vi "pointReactorSimulator.vi"() -> ()   [LabVIEW 2020]
doc: "本程序通过点堆动力学模型模拟核电站的反应堆运行状态。"
uses:
  <vilib>/Utility/sysdir.llb/System Directory Type.ctl
  <vilib>/NI/Modbus Library/API/Slave/Modbus Slave.lvclass
  <vilib>/Utility/error.llb/DialogType.ctl
  Keithley 622x/Utility/Typedefs/KE622x -- Instrument Type.ctl
  Keithley 622x/Configure/Source/Typedefs/KE622x -- Voltage Limit.ctl
  Keithley 622x/Configure/Source/Typedefs/KE622x -- Current Range.ctl
  Keithley 622x/Configure/Source/Typedefs/KE622x -- Current Ranges.ctl
  <vilib>/DAQmx/write.llb/DAQmx Write (Counter 1D Frequency 1Chan NSamp).vi
  <vilib>/DAQmx/write.llb/DAQmx Write (Analog DBL 1Chan 1Samp).vi
  SettingVariable.vi
  <vilib>/Utility/file.llb/Read Delimited Spreadsheet (DBL).vi
  <userlib>/_OpenG.lib/array/array.llb/Reverse 2D Array (DBL)__ogtk.vi
  <vilib>/Analysis/polynomials.llb/Scalar Polynomial Evaluation (DBL).vi
  <vilib>/NI/Modbus Library/API/Wrapper/Create TCP Slave.vi
  <vilib>/Instr/_visa.llb/VISA Configure Serial Port (Instr).vi
  <vilib>/DAQmx/create/channels.llb/DAQmx Create Channel (CO-Pulse Generation-Frequency).vi
  <vilib>/DAQmx/configure/timing.llb/DAQmx Timing (Implicit).vi
  <vilib>/DAQmx/create/channels.llb/DAQmx Create Channel (AO-Voltage-Basic).vi
  <vilib>/DAQmx/miscellaneous.llb/DAQmx Fill In Error Info.vi
  PointReactorDll.dll
  <vilib>/Analysis/NI_AALPro.lvlib
  Keithley 622x/Keithley 622x.lvlib
  <vilib>/NI/Modbus Library/API/Wrapper/API Main.lvlib
panel:
  in  "退出":bool
  out "KE6220_2":bool
  in  "物理参数设置":bool
  out "反应性仪输出电压":dbl[](array[numeric])
  out "输出电压":dbl[](array[numeric])
  in  "输出电流 (A)":dbl
  in  "电压输出选择":bool
  out "中子注量率":dbl caption="(n/cm2·s)"
  out "硼总价值 (pcm)":dbl
  out "棒总价值 (pcm)":dbl
  out "硼浓度 indicator":dbl
  in  "硼浓度 (ppm)":dbl(slide)=1.0 scale=0.0..2000.0
  out "运行时间":dbl caption="(s)"
  in  "TCP端口号":u16=502 caption="TCP端口号：" min=1 max=9999
  out "堆芯反应性(硼+棒) (pcm)":dbl
  out "keff":dbl
  in  "S棒组":dbl(slide)=200.0 min=0.0 max=225.0 scale=0.0..225.0
  in  "A棒组":dbl(slide)=200.0 min=0.0 max=225.0 scale=0.0..225.0
  in  "B棒组":dbl(slide)=200.0 min=0.0 max=225.0 scale=0.0..225.0
  in  "C棒组":dbl(slide)=200.0 min=0.0 max=225.0 scale=0.0..225.0
  in  "堆芯后备反应性 (pcm)":dbl
  out "S棒价值":dbl
  out "A棒价值":dbl
  out "B棒价值":dbl
  out "C棒价值":dbl
  out "D棒价值":dbl
  out "中子注量曲线":dbl(graph) caption="波形图"
  in  "D棒组":dbl(slide)=200.0 min=0.0 max=225.0 scale=0.0..225.0
  out "CARD":bool
  out "KE6220_1":bool
  out "COM2":bool
  out "COM1":bool
  in  "VO 4":u16(ring)=3 items=["D棒位 (step)", "C棒位 (step)", "B棒位 (step)", "A棒位 (step)", "S棒位 (step)", "硼浓度 (ppm)", "中间量程电流 (A)", "源量程计数 (CPS)"]
  in  "VO 3":u16(ring)=2 items=["D棒位 (step)", "C棒位 (step)", "B棒位 (step)", "A棒位 (step)", "S棒位 (step)", "硼浓度 (ppm)", "中间量程电流 (A)", "源量程计数 (CPS)"]
  in  "VO 2":u16(ring)=1 items=["D棒位 (step)", "C棒位 (step)", "B棒位 (step)", "A棒位 (step)", "S棒位 (step)", "硼浓度 (ppm)", "中间量程电流 (A)", "源量程计数 (CPS)"]
  in  "VO 1":u16(ring) items=["D棒位 (step)", "C棒位 (step)", "B棒位 (step)", "A棒位 (step)", "S棒位 (step)", "硼浓度 (ppm)", "中间量程电流 (A)", "源量程计数 (CPS)"]
  in  "电信号输出设置":bool
  in  "TCP服务器开关":bool caption="TCP服务器开："
  in  "电流输出选择":u16(ring) items=["中间量程电流", "功率量程电流"]
  out "棒位与硼浓度":dbl[](array[numeric])
  in  "反应性控制方式":bool
  in  "归零":bool
  in  "棒速(step/min)":dbl=72.0 min=1.0 max=10000.0 step=1.0 format="%#.3g"
  in  "开始降棒":bool
  in  "降棒选择":u16(ring) items=["D棒组", "C棒组", "B棒组", "A棒组", "S棒组"]
  in  "细分时间 (ms)":u32=100 min=10 max=1000 step=1
  in  "开始":bool
  in  "时间比例尺":dbl(knob)=1.0 min=0.1 max=1000.0 step=0.1 scale=0.1..1000.0
  out "功率量程 (A)":dbl(slide) scale=2.875e-12..0.00023 scale format="%#_6e"
  out "中间量程 (A)":dbl(slide) scale=1e-11..0.0008 scale format="%#_6e"
  out "源量程 (CPS)":dbl(slide) scale=1.0..1000000.0 scale format="%#_6f"
  out "%FP":dbl(slide) scale=2e-09..200.0 scale format="%#_6e"
  out "中子注量率":dbl(slide) scale=0.1..10000000000.0 scale format="%#_6e"
  in  "时间步长":dbl=0.1 caption="时间步长："
  in  "初始注量率":dbl=1000.0 caption="初始注量率：" format="%#_4g"
  in  "堆芯反应性":dbl caption="堆芯反应性 (pcm)"
  in  "停止":bool
  # "反应性仪测试用点堆模拟器"
  # "探测器"
  # "手输"
  # "棒硼"
  # "1.25E+5 n/cm2·s\n——"
  # "——\n1.25E+2 n/cm2·s"
  # "——  1.25E-1 n/cm2·s"
  # "(n/cm2·s)"
  # "硬件测试"
  # "(s)"
  # "0-10V"
  # "1-5V"
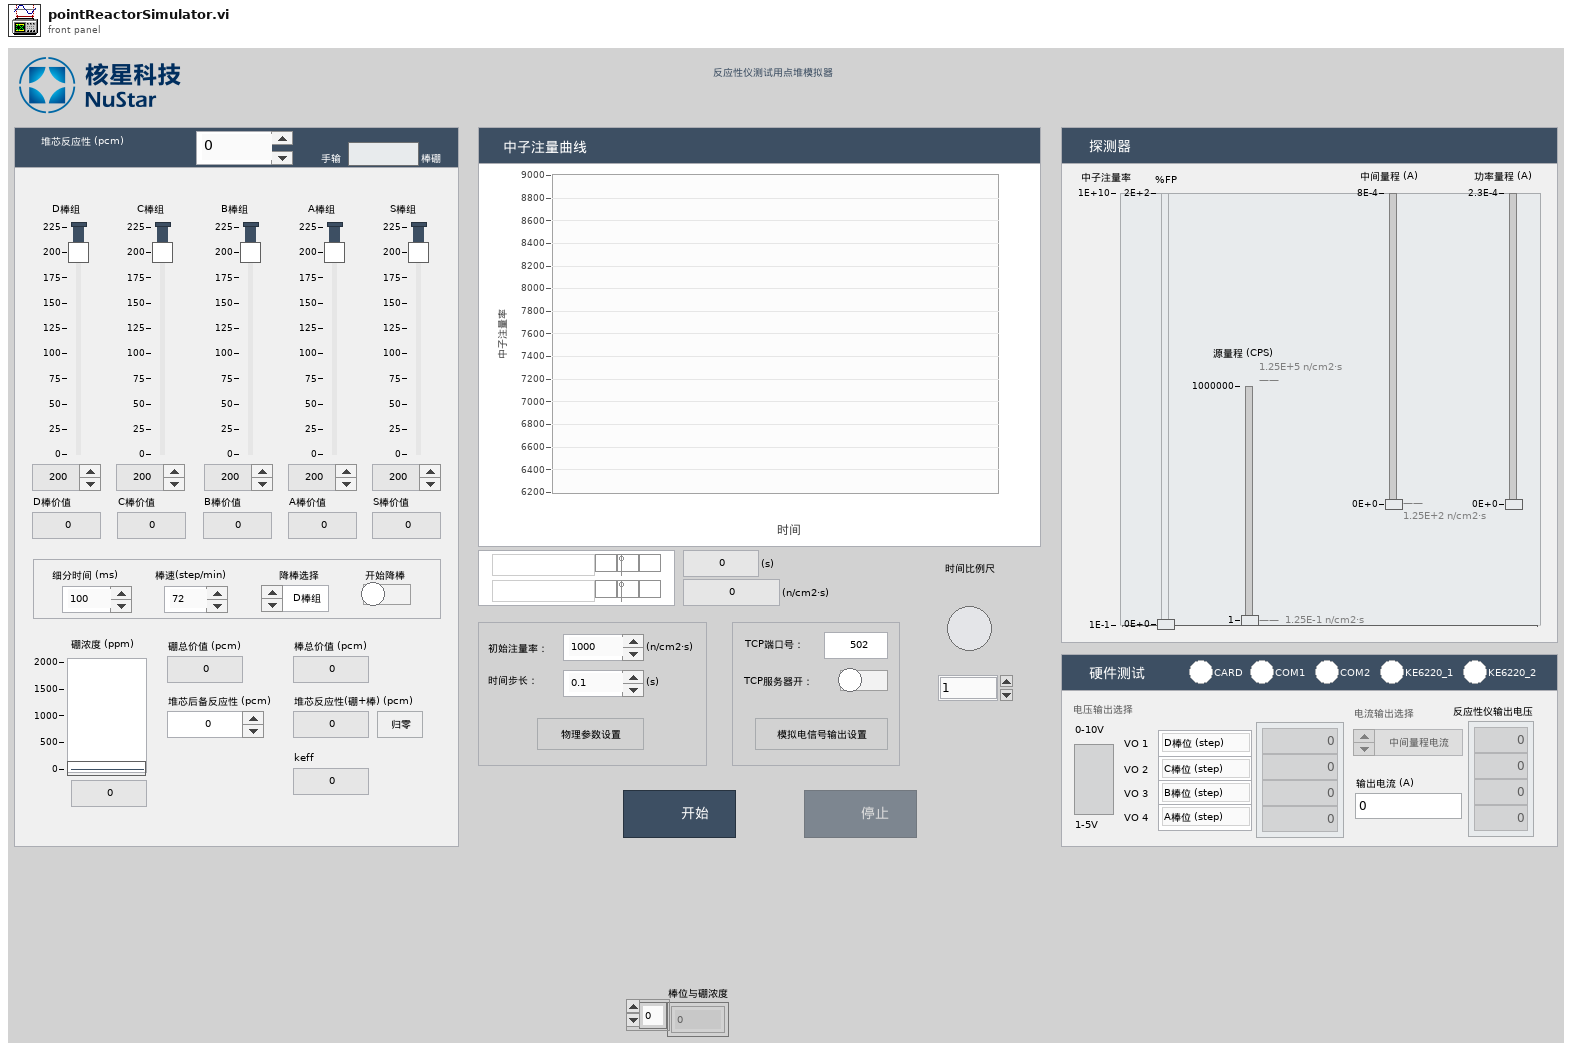
[diagram p1: front panel]
types:
  T1 = enum8{"Enabled", "Disabled", "Disabled and Grayed Out"}
  T2 = enum16{"open", "replace", "create", "open or create", "replace or create", "replace or create with confirmation"}
  T3 = typedef "Keithley 622x.lvlib/KE622x -- Voltage Limit.ctl" = dbl
  T4 = typedef "Keithley 622x.lvlib/KE622x -- Instrument Type.ctl" = enum16{"KE6220", "KE6221"}
  T5 = typedef "System Directory Type.ctl" = i32
  T6 = typedef "DialogType.ctl" = u16
  T7 = typedef "Keithley 622x.lvlib/KE622x -- Current Range.ctl" = cluster{"Auto Range?":bool, "Man / Selected\nRange":T8}
  T8 = typedef "Keithley 622x.lvlib/KE622x -- Current Ranges.ctl" = enum16{"2nA", "20nA", "200nA", "2uA", "20uA", "200uA", "2mA", "20mA", "100mA"}
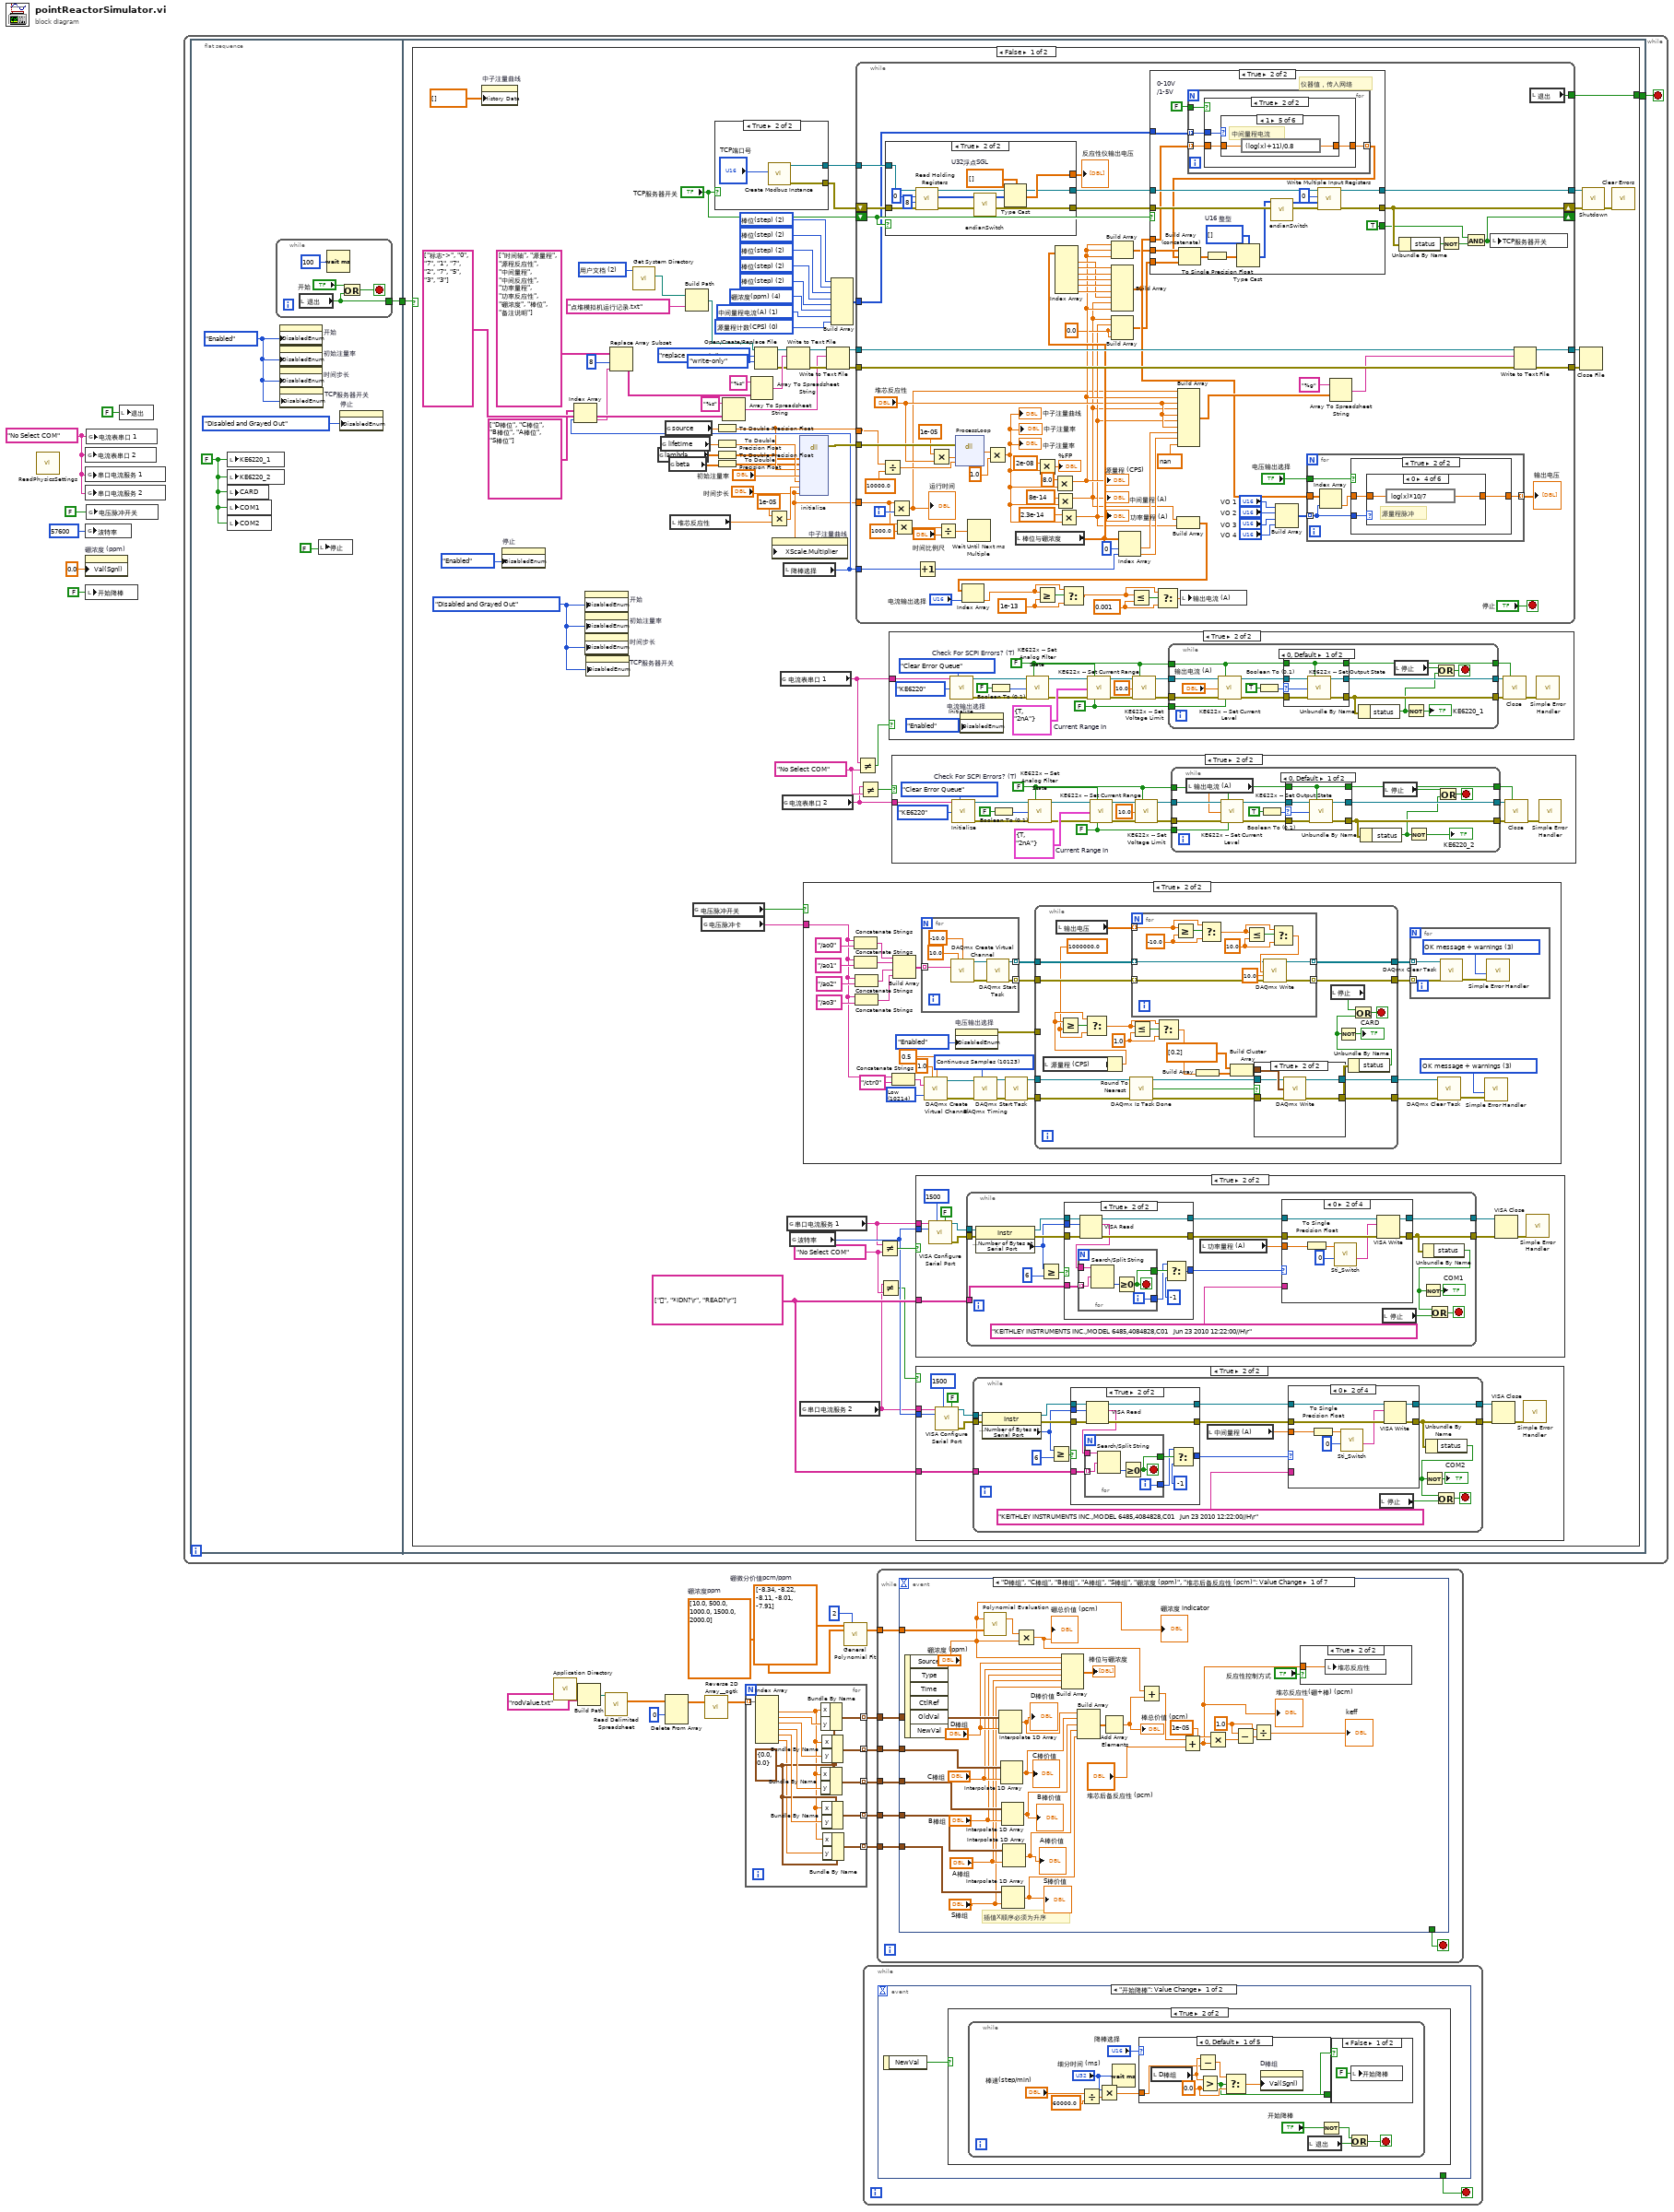
[diagram p0: block diagram]
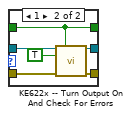
[diagram p3: hidden frame]
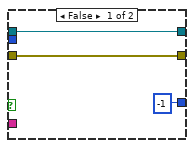
[diagram p5: hidden frame]
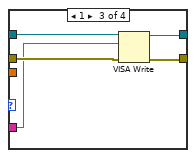
[diagram p7: hidden frame]
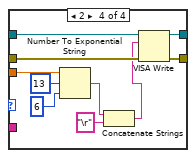
[diagram p8: hidden frame]
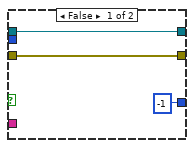
[diagram p10: hidden frame]
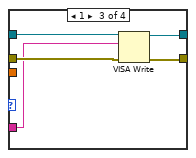
[diagram p12: hidden frame]
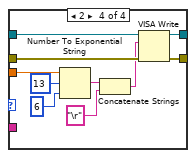
[diagram p13: hidden frame]
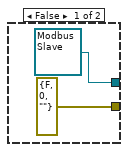
[diagram p14: hidden frame]
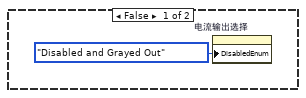
[diagram p15: hidden frame]
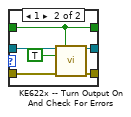
[diagram p16: hidden frame]
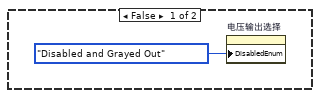
[diagram p17: hidden frame]
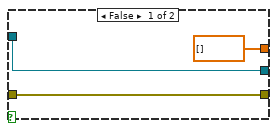
[diagram p19: hidden frame]
diagram:
  w12 = "No Select COM" ("新元素/子数组")
  w20 = dbl[] [-8.34, -8.22, -8.11, -8.01, -7.91]  # 硼微分价值pcm/ppm
  w19 = dbl[] [10.0, 500.0, 1000.0, 1500.0, 2000.0]  # 硼浓度ppm
  n1 = call "ReadPhysicsSettings.vi"() -> ()  [unwired: 12 in]
  n2 = property on="硼浓度 (ppm)" class="Slide (strict)"("Val(Sgnl)"=0.0 ("Value (Signaling)")) -> ()  [unwired: 2 in, 2 out]
  n3 = global write "SettingVariable.vi" "电流表串口 2"(w12) -> ()
  n4 = global write "SettingVariable.vi" "串口电流服务 1"(w12) -> ()
  n5 = global write "SettingVariable.vi" "串口电流服务 2"(w12) -> ()
  n6 = global write "SettingVariable.vi" "波特率"(u32 57600 ("波特率")) -> ()
  n7 = local write "开始降棒"(FALSE ("开始降棒")) -> ()
  n8 = global write "SettingVariable.vi" "电流表串口 1"(w12) -> ()
  n9 = global write "SettingVariable.vi" "电压脉冲开关"(FALSE ("电压脉冲开关")) -> ()
  n10 = local write "退出"(FALSE ("退出")) -> ()
  n11 = while {
    stop <- w24 stop-if-true
    n12 = flat-sequence {
      tunnel: [w26] -> w23
      tunnel: [w35] -> w24
      tunnel: w23 -> [w34]
      frame #0 {
        w29 = FALSE ("KE6220_1")
        w25 = T1."Enabled" ("禁用")
        n13 = local write "KE6220_1"(w29) -> ()
        n14 = local write "KE6220_2"(w29) -> ()
        n15 = local write "CARD"(w29) -> ()
        n16 = local write "COM1"(w29) -> ()
        n17 = local write "COM2"(w29) -> ()
        n18 = while {
          tunnel: [w30] -> w26
          stop <- w32 stop-if-true
          n19 = local read "退出"() -> (w30:bool)
          n20 = Wait (ms)(milliseconds to wait=u32 100) -> ()  [unwired: 1 out]
          n21 = Or(x="开始", y=w30) -> (x .or. y?=w32:bool)
        }
        n22 = property on="开始" class="Bool"("DisabledEnum"=w25) -> ()  [unwired: 2 in, 2 out]
        n23 = property on="初始注量率" class="DigNum (strict)"("DisabledEnum"=w25) -> ()  [unwired: 2 in, 2 out]
        n24 = property on="时间步长" class="DigNum (strict)"("DisabledEnum"=w25) -> ()  [unwired: 2 in, 2 out]
        n25 = property on="TCP服务器开关" class="Bool (strict)"("DisabledEnum"=w25) -> ()  [unwired: 2 in, 2 out]
        n26 = local write "停止"(FALSE ("退出")) -> ()
        n27 = property on="停止" class="Bool (strict)"("DisabledEnum"=T1."Disabled and Grayed Out" ("禁用")) -> ()  [unwired: 2 in, 2 out]
      }
      frame #1 {
        n28 = case shown="False" w34 {
          tunnel: [w47 TRUE ("退出")] -> w35
          frame False {
            w36 = T1."Disabled and Grayed Out" ("禁用")
            w67 = u16 0 items=["源量程计数(CPS)", "中间量程电流(A)", "棒位(step)", "温度(℃)", "硼浓度(ppm)", "P2电压信号"] ("P2-1")
            w68 = u16 1 items=["源量程计数(CPS)", "中间量程电流(A)", "棒位(step)", "温度(℃)", "硼浓度(ppm)", "P2电压信号"] ("P2-1")
            w69 = u16 4 items=["源量程计数(CPS)", "中间量程电流(A)", "棒位(step)", "温度(℃)", "硼浓度(ppm)", "P2电压信号"] ("P2-1")
            w70 = u16 2 items=["源量程计数(CPS)", "中间量程电流(A)", "棒位(step)", "温度(℃)", "硼浓度(ppm)", "P2电压信号"] ("P2-1")
            w71 = u16 2 items=["源量程计数(CPS)", "中间量程电流(A)", "棒位(step)", "温度(℃)", "硼浓度(ppm)", "P2电压信号"] ("P2-1")
            w72 = u16 2 items=["源量程计数(CPS)", "中间量程电流(A)", "棒位(step)", "温度(℃)", "硼浓度(ppm)", "P2电压信号"] ("P2-1")
            w73 = u16 2 items=["源量程计数(CPS)", "中间量程电流(A)", "棒位(step)", "温度(℃)", "硼浓度(ppm)", "P2电压信号"] ("P2-1")
            w57 = "No Select COM" ("新元素/子数组")
            w79 = T5 2 items=["用户目录"=0, "用户桌面"=1, "用户文档"=2, "用户应用程序数据"=3, "用户设置"=4, "用户临时目录"=5, "公共文档"=6, "公共应用程序数据"=7, "公共设置"=8, "公共缓存"=13, "系统核心库"=9, "系统安装库"=10, "应用程序文件"=11, "启动盘根目录"=12] ("system directory type")
            w81 = "No Select COM" ("新元素/子数组")
            w83 = string[] ["", "*IDN?\r", "READ?\r"] ("添加的数组")
            w85 = u16 2 items=["源量程计数(CPS)", "中间量程电流(A)", "棒位(step)", "温度(℃)", "硼浓度(ppm)", "P2电压信号"] ("P2-1")
            n29 = property on="中子注量曲线" class="WFChart (strict)"("History Data"=dbl[] []) -> ()  [unwired: 2 in, 2 out]
            n30 = property on="停止" class="Bool (strict)"("DisabledEnum"=T1."Enabled" ("禁用")) -> ()  [unwired: 2 in, 2 out]
            n31 = property on="开始" class="Bool"("DisabledEnum"=w36) -> ()  [unwired: 2 in, 2 out]
            n32 = property on="初始注量率" class="DigNum (strict)"("DisabledEnum"=w36) -> ()  [unwired: 2 in, 2 out]
            n33 = property on="时间步长" class="DigNum (strict)"("DisabledEnum"=w36) -> ()  [unwired: 2 in, 2 out]
            n34 = property on="TCP服务器开关" class="Bool (strict)"("DisabledEnum"=w36) -> ()  [unwired: 2 in, 2 out]
            n35 = call <vilib>:"Get System Directory.vi"("system directory type"=w79) -> ("system directory"=w80:path)  [unwired: 10 in]
            n36 = global read "SettingVariable.vi" "lambda"() -> (w49:dbl[])
            n37 = global read "SettingVariable.vi" "lifetime"() -> (w52:dbl)
            n38 = global read "SettingVariable.vi" "source"() -> (w51:dbl)
            n39 = global read "SettingVariable.vi" "beta"() -> (w50:dbl[])
            n40 = local read "堆芯反应性"() -> (w45:dbl)
            n41 = Build Path(base path=w80, name or relative path="点堆模拟机运行记录.txt") -> (appended path=w41:path)
            n42 = global read "SettingVariable.vi" "电压脉冲开关"() -> (w61:bool)
            n43 = global read "SettingVariable.vi" "电压脉冲卡"() -> (w60:tag)
            n44 = case shown="True" "TCP服务器开关" {
              tunnel: [errorcluster {"status"=FALSE, "code"=0, "source"=""} ("error out") w306] -> w87
              tunnel: [refnum<class "Modbus Slave.lvclass"> refnum ("TCP slave instance") w305] -> w66
              frame False {
              }
              frame True {
                n45 = call-poly <vilib>:"Create Modbus Instance.vi"("port (502)"="TCP端口号") -> ("error out"=w306:errorcluster, "TCP slave instance"=w305:refnum<class "Modbus Slave.lvclass">)  [unwired: 9 in]
              }
            }
            n46 = To Double Precision Float(number=w51) -> (double precision float=w76:dbl)
            n47 = To Double Precision Float(number=w52) -> (double precision float=w77:dbl)
            n48 = To Double Precision Float(number=w49) -> (double precision float=w74:dbl[])
            n49 = To Double Precision Float(number=w50) -> (double precision float=w75:dbl[])
            n50 = Array To Spreadsheet String(array=string[] ["标志->", "0", "7", "1", "7", "2", "7", "5", "3", "3"] ("添加的数组"), 3:"%s" ("format string")) -> (spreadsheet string=w100:string)  [unwired: 1 in]
            n51 = Open/Create/Replace File(file path (use dialog)=w41, operation (0:open)=T2."replace or create", access (0:read/write)=enum16{"read/write", "read-only", "write-only"}."write-only") -> (refnum out=w40:refnum<file>, error out=w39:errorcluster)  [unwired: 3 in, 1 out]
            n52 = Multiply(x=1e-05, y=w45) -> (x*y=w94:dbl)
            n53 = property on="中子注量曲线" class="WFChart (strict)"("XScale.Multiplier"="时间步长") -> ()  [unwired: 2 in, 2 out]
            n54 = global read "SettingVariable.vi" "电流表串口 1"() -> (w59:string)
            n55 = global read "SettingVariable.vi" "电流表串口 2"() -> (w56:string)
            n56 = local read "降棒选择"() -> (w88:u16)
            n57 = Index Array(array=string[] ["D棒位", "C棒位", "B棒位", "A棒位", "S棒位"] ("添加的数组"), index=w88) -> (element=w91:string)
            n58 = Replace Array Subset(array=string[] ["时间轴", "源量程", "源程反应性", "中间量程", "中间反应性", "功率量程", "功率反应性", "硼浓度", "棒位", "备注说明"] ("添加的数组"), new element=w91, index=8 ("索引")) -> (w90:string[])
            n59 = Array To Spreadsheet String(array=w90, 3:"%s" ("format string")) -> (spreadsheet string=w104:string)  [unwired: 1 in]
            n60 = Write to Text File(file (use dialog)=w40, text=w104, error in=w39) -> (refnum out=w103:refnum<file>, error out=w102:errorcluster)  [unwired: 1 in, 1 out]
            n61 = global read "SettingVariable.vi" "串口电流服务 1"() -> (w55:string)
            n62 = global read "SettingVariable.vi" "波特率"() -> (w62:u32)
            n63 = dll-call lib="D:/LVprojects/PointReactorSimulator/src/PointReactorDll.dll" fn="initialize"("lamd"=w74, "bet"=w75, "source"=w76, "n0"="初始注量率", "nlife"=w77, "reactivity"=w94, "delt"="时间步长") -> (error out=w107:errorcluster)  [unwired: 3 in, 9 out]
            n64 = global read "SettingVariable.vi" "串口电流服务 2"() -> (w53:string)
            n65 = case shown="True" w61 {
              tunnel: w60 -> [_ w360]
              frame False {
                n66 = property on="电压输出选择" class="Bool (strict)"("DisabledEnum"=T1."Disabled and Grayed Out" ("禁用")) -> ()  [unwired: 2 in, 2 out]
              }
              frame True {
                w377 = 10214 items=["High"=10192, "Low"=10214] ("Idle State")
                w376 = 10123 items=["Finite Samples"=10178, "Continuous Samples"=10123] ("sample mode")
                w381 = T6 3 items=["no dialog", "OK message", "continue or stop message", "OK message + warnings", "continue/stop + warnings"] ("type of dialog (OK msg:1)")
                n67 = Concatenate Strings(w360, "/ao0") -> (w365:string)
                n68 = Concatenate Strings(w360, "/ao1") -> (w364:string)
                n69 = Concatenate Strings(w360, "/ao2") -> (w363:string)
                n70 = Concatenate Strings(w360, "/ao3") -> (w362:string)
                n71 = Concatenate Strings(w360, "/ctr0") -> (w369:string)
                n72 = Build Array(w365, w364, w363, w362) -> (w361:string[])
                n73 = for {
                  tunnel: [w398] -> w387 mode=indexing
                  tunnel: [w397] -> w386 mode=indexing
                  tunnel: w361 -> [w396] mode=indexing
                  n74 = call-poly <vilib>:"DAQmx Create Virtual Channel.vi"("maximum value"=10.0 ("Maximum Value"), "minimum value"=-10.0 ("Minimum Value"), "physical channels"=w396) -> ("task out"=w400:refnum<k21>, "error out"=w399:errorcluster)  [unwired: 11 in]
                  n75 = call <vilib>:"DAQmx Start Task.vi"("task/channels in"=w400, "error in"=w399) -> ("task out"=w398:refnum<k21>, "error out"=w397:errorcluster)  [unwired: 12 in]
                }
                n76 = call-poly <vilib>:"DAQmx Create Virtual Channel.vi"("frequency"=1.0 ("duty cycle"), "duty cycle"=0.5, "counter"=w369, "idle state"=w377) -> ("task out"=w373:refnum<k21>, "error out"=w372:errorcluster)  [unwired: 10 in]
                n77 = property on="电压输出选择" class="Bool (strict)"("DisabledEnum"=T1."Enabled" ("禁用")) -> (error out=w384:errorcluster)  [unwired: 2 in, 1 out]
                n78 = call-poly <vilib>:"DAQmx Timing.vi"("task/channels in"=w373, "sample mode"=w376, "error in"=w372) -> ("task out"=w375:refnum<k21>, "error out"=w374:errorcluster)  [unwired: 11 in]
                n79 = call <vilib>:"DAQmx Start Task.vi"("task/channels in"=w375, "error in"=w374) -> ("task out"=w371:refnum<k21>, "error out"=w370:errorcluster)  [unwired: 12 in]
                n80 = while {
                  tunnel: [w429] -> w390
                  tunnel: [w428] -> w389
                  tunnel: w387 -> [w427]
                  tunnel: w386 -> [w426]
                  tunnel: [w417] -> w383
                  tunnel: [w413] -> w382
                  tunnel: w371 -> [w408]
                  tunnel: w384 -> [_]
                  tunnel: w370 -> [w407]
                  stop <- w410 stop-if-true
                  w419 = 1000000.0 ("y")
                  w422 = 1.0 ("y")
                  n81 = local read "源量程 (CPS)"() -> (w425:dbl)
                  n82 = local read "输出电压"() -> (w403:dbl[])
                  n83 = Round To Nearest(number=w425) -> (nearest integer value=w420:dbl)
                  n84 = Greater Or Equal?(x=w420, y=w419) -> (x >= y?=w424:bool)
                  n85 = Select(t=w420, s=w424, f=w419) -> (s? t:f=w421:dbl)
                  n86 = call <vilib>:"DAQmx Is Task Done.vi"("task/channels in"=w408, "error in"=w407) -> ("task out"=w406:refnum<k21>, "task done?"=w404:bool, "error out"=w405:errorcluster)  [unwired: 11 in]
                  n87 = Less Or Equal?(x=w421, y=w422) -> (x <= y?=w423:bool)
                  n88 = for {
                    tunnel: [w447] -> w429 mode=indexing
                    tunnel: [w446] -> w428 mode=indexing
                    tunnel: w427 -> [w439] mode=indexing
                    tunnel: w426 -> [w438] mode=indexing
                    tunnel: w403 -> [w437] mode=indexing
                    w442 = 10.0 ("y")
                    w444 = -10.0 ("y")
                    n89 = Greater Or Equal?(x=w437, y=w444) -> (x >= y?=w445:bool)
                    n90 = Select(t=w437, s=w445, f=w444) -> (s? t:f=w441:dbl)
                    n91 = Less Or Equal?(x=w441, y=w442) -> (x <= y?=w443:bool)
                    n92 = Select(t=w441, s=w443, f=w442) -> (s? t:f=w440:dbl)
                    n93 = call-poly <vilib>:"DAQmx Write.vi"("task/channels in"=w439, "data"=w440, "timeout"=10.0, "error in"=w438) -> ("task out"=w447:refnum<k21>, "error out"=w446:errorcluster)  [unwired: 9 in, 1 out]
                  }
                  n94 = Select(t=w421, s=w423, f=w422) -> (s? t:f=w414:dbl)
                  n95 = Build Array(w414) -> (w415:dbl[])
                  n96 = Build Cluster Array(dbl[] [0.2] ("数组"), w415) -> (w418:cluster{"initial delay":dbl, "y":dbl}[])
                  n97 = case shown="True" w404 {
                    tunnel: w418 -> [_ w436]
                    tunnel: [w431 w435] -> w417
                    tunnel: [w430 w434] -> w413
                    tunnel: w406 -> [w431 w433]
                    tunnel: w405 -> [w430 w432]
                    frame False {
                    }
                    frame True {
                      n98 = call-poly <vilib>:"DAQmx Write.vi"("task/channels in"=w433, "data"=w436, "error in"=w432) -> ("task out"=w435:refnum<k21>, "error out"=w434:errorcluster)  [unwired: 10 in, 1 out]
                    }
                  }
                  n99 = local read "停止"() -> (w409:bool)
                  n100 = Unbundle By Name(w413) -> ("status"=w411:bool)
                  n101 = Not(x=w411) -> (.not. x?=→"CARD":bool)
                  n102 = Or(x=w409, y=w411) -> (x .or. y?=w410:bool)
                }
                n103 = for {
                  tunnel: w390 -> [w393] mode=indexing
                  tunnel: w389 -> [w392] mode=indexing
                  w394 = T6 3 items=["no dialog", "OK message", "continue or stop message", "OK message + warnings", "continue/stop + warnings"] ("type of dialog (OK msg:1)")
                  n104 = call <vilib>:"DAQmx Clear Task.vi"("task in"=w393, "error in"=w392) -> ("error out"=w395:errorcluster)  [unwired: 13 in]
                  n105 = call <vilib>:"Simple Error Handler.vi"("type of dialog (OK msg:1)"=w394, "error in (no error)"=w395) -> ()  [unwired: 3 in, 5 out]
                }
                n106 = call <vilib>:"DAQmx Clear Task.vi"("task in"=w383, "error in"=w382) -> ("error out"=w380:errorcluster)  [unwired: 13 in]
                n107 = call <vilib>:"Simple Error Handler.vi"("type of dialog (OK msg:1)"=w381, "error in (no error)"=w380) -> ()  [unwired: 3 in, 5 out]
              }
            }
            n108 = Write to Text File(file (use dialog)=w103, text=w100, error in=w102) -> (refnum out=w98:refnum<file>, error out=w97:errorcluster)  [unwired: 1 in, 1 out]
            n109 = Build Array(w85, w73, w72, w71, w70, w69, w68, w67) -> (w84:u16[])
            n110 = while {
              tunnel: w107 -> [w527]
              tunnel: "时间步长" -> [w506]
              tunnel: w98 -> [w524]
              tunnel: w97 -> [w523]
              tunnel: [w522] -> w38
              tunnel: [w521] -> w37
              tunnel: w76 -> [w505]
              tunnel: w88 -> [w457]
              tunnel: w84 -> [w454]
              tunnel: w66 -> [w462]
              tunnel: [w460] -> w64
              shift-right: [w475] -> w65
              shift-left: w87 -> [w471]
              tunnel: [w459] -> w47
              shift-right: [w456] -> _
              shift-left: "TCP服务器开关" -> [w469]
              i -> [w526]
              stop <- "停止" stop-if-true
              w468 = 0.0 ("元素")
              w495 = 0.001 ("y")
              w498 = 1e-13 ("y")
              n111 = Divide(x=w505, y=10000.0) -> (x/y=w504:dbl)
              n112 = case shown="True" w469 {
                tunnel: w471 -> [w531 w541]
                tunnel: [w531 w540] -> w470
                tunnel: [sgl[] [] ("单精度浮点") w538] -> w464
                tunnel: w462 -> [w529 w535]
                tunnel: [w529 w534] -> w461
                frame False {
                }
                frame True {
                  w539 = sgl[] []  # U32浮点SGL
                  n113 = call-dynamic "Read Holding Registers.vi"("error in"=w541, "number of inputs"=u16 8 ("Quantity"), "starting address"=u16 0 ("Address"), "Modbus slave in"=w535) -> ("error out"=w540:errorcluster, "register values"=w532:u16[], "Modbus slave out"=w534:refnum<class "Modbus Slave.lvclass">)  [unwired: 5 in]
                  n114 = call "endianSwitch.vi"("U16 array in"=w532) -> ("U16 array out"=w533:u16[])  [unwired: 10 in]
                  n115 = Type Cast(type=w539, x=w533) -> (*(type *) &x=w538:sgl[])
                }
              }
              "反应性仪输出电压" <- w464
              n116 = Multiply(x=w506, y=w526) -> (x*y=w449:dbl)
              "运行时间" <- w449
              n117 = Multiply(x=w506, y=1000.0) -> (x*y=w508:dbl)
              n118 = Increment(x=w457) -> (x+1=w458:u16)
              n119 = Multiply(x=1e-05, y="堆芯反应性") -> (x*y=w518:dbl)
              n120 = Divide(x=w508, y="时间比例尺") -> (x/y=w450:dbl)
              n121 = dll-call lib="D:/LVprojects/PointReactorSimulator/src/PointReactorDll.dll" fn="ProcessLoop"(error in=w527, "reactivity"=w518, "nmin"=w504) -> ("nflux"=w511:dbl)  [unwired: 2 in, 4 out]
              n122 = Wait Until Next ms Multiple(millisecond multiple=w450) -> ()  [unwired: 1 out]
              n123 = Multiply(x=w511, y=1.0) -> (x*y=w451:dbl)
              "中子注量率" <- w451
              "中子注量曲线" <- w451
              "中子注量率" <- w451
              n124 = local read "棒位与硼浓度"() -> (w489:dbl[])
              n125 = Multiply(x=2e-08 ("y"), y=w451) -> (x*y=→"%FP":dbl)
              n126 = Multiply(x=8.0 ("y"), y=w451) -> (x*y=w481:dbl)
              "源量程 (CPS)" <- w481
              n127 = Multiply(x=8e-14 ("y"), y=w451) -> (x*y=w466:dbl)
              "中间量程 (A)" <- w466
              n128 = Index Array(array=w489) -> (element #1=w483:dbl, element #2=w488:dbl, element #3=w487:dbl, element #4=w486:dbl, element #5=w485:dbl, element #6=w484:dbl)  [unwired: 6 in]
              n129 = Multiply(x=2.3e-14 ("y"), y=w451) -> (x*y=w467:dbl)
              "功率量程 (A)" <- w467
              n130 = Build Array(w481, w481, w481) -> (w453:dbl[])
              n131 = Build Array(w488, w487, w486, w485, w484, w483, w466, w481) -> (w455:dbl[])
              n132 = Build Array(w466, w467, w468, w468) -> (w452:dbl[])
              n133 = Index Array(array=w489, index #1=0 ("索引"), index #2=w458) -> (element #1=w492:dbl, element #2=w491:dbl)
              n134 = case shown="True" w469 {
                tunnel: w470 -> [w575 w591]
                tunnel: [w575 w590] -> w475
                tunnel: [FALSE TRUE] -> w472
                tunnel: w461 -> [w573 w588]
                tunnel: [w573 w587] -> w460
                tunnel: w455 -> [_ w586]
                tunnel: w454 -> [_ w584]
                tunnel: w453 -> [_ w582]
                tunnel: w452 -> [_ w581]
                frame False {
                }
                frame True {
                  w583 = u16[] []  # U16 整型
                  w585 = FALSE  # 0-10V /1-5V
                  # "仪器值，传入网络"
                  n135 = for {
                    tunnel: w586 -> [w595] mode=indexing
                    tunnel: [w594] -> w580 mode=indexing
                    tunnel: w585 -> [w596]
                    tunnel: w584 -> [w593] mode=indexing
                    n136 = case shown="True" w596 {
                      tunnel: w595 -> [w599 w613]
                      tunnel: [w598 w612] -> w594
                      tunnel: w593 -> [w597 w611]
                      frame False {
                        n137 = case shown="4" w597 {
                          tunnel: w599 -> [w601 w603 w604 w606 w607 w610]
                          tunnel: [w600 w602 w604 w605 w608 w609] -> w598
                          frame 3 {
                            # "温度"
                            n138 = expression code="(x-275) *4/60+1"(w601) -> (w600:dbl)
                          }
                          frame 4 {
                            # "硼浓度"
                            n139 = expression code="x*4/2000+1"(w603) -> (w602:dbl)
                          }
                          frame Default {
                          }
                          frame 0 {
                            # "源量程脉冲"
                            n140 = expression code="log(x)*4/7+1"(w606) -> (w605:dbl)
                          }
                          frame 1 {
                            # "中间量程电流"
                            n141 = expression code="(log(x)+11)/2+1"(w607) -> (w608:dbl)
                          }
                          frame 2 {
                            # "棒位"
                            n142 = expression code="x*4/225+1"(w610) -> (w609:dbl)
                          }
                        }
                      }
                      frame True {
                        n143 = case shown="1" w611 {
                          tunnel: w613 -> [w615 w617 w618 w620 w621 w623]
                          tunnel: [w614 w616 w618 w619 w622 w624] -> w612
                          frame 3 {
                            # "温度"
                            n144 = expression code="(x-275)*10/60"(w615) -> (w614:dbl)
                          }
                          frame 4 {
                            # "硼浓度"
                            n145 = expression code="x*10/2000"(w617) -> (w616:dbl)
                          }
                          frame Default {
                          }
                          frame 0 {
                            # "源量程脉冲"
                            n146 = expression code="log(x)*10/7"(w620) -> (w619:dbl)
                          }
                          frame 1 {
                            # "中间量程电流"
                            n147 = expression code="(log(x)+11)/0.8"(w621) -> (w622:dbl)
                          }
                          frame 2 {
                            # "棒位"
                            n148 = expression code="10*x/225"(w623) -> (w624:dbl)
                          }
                        }
                      }
                    }
                  }
                  n149 = Build Array (concatenate)(w582, w580, w581) -> (w578:dbl[])
                  n150 = To Single Precision Float(number=w578) -> (single precision float=w579:sgl[])
                  n151 = Type Cast(type=w583, x=w579) -> (*(type *) &x=w577:u16[])
                  n152 = call "endianSwitch.vi"("U16 array in"=w577) -> ("U16 array out"=w576:u16[])  [unwired: 10 in]
                  n153 = call-dynamic "Write Multiple Input Registers.vi"("error in"=w591, "input registers to write"=w576, "starting address"=u16 0 ("Address"), "Modbus slave in"=w588) -> ("error out"=w590:errorcluster, "Modbus slave out"=w587:refnum<class "Modbus Slave.lvclass">)  [unwired: 6 in]
                }
              }
              n154 = Build Array(w466, w467) -> (w501:dbl[])
              n155 = Index Array(array=w501, index="电流输出选择") -> (element=w497:dbl)
              n156 = Greater Or Equal?(x=w497, y=w498) -> (x >= y?=w499:bool)
              n157 = Select(t=w497, s=w499, f=w498) -> (s? t:f=w494:dbl)
              n158 = Less Or Equal?(x=w494, y=w495) -> (x <= y?=w496:bool)
              n159 = Select(t=w494, s=w496, f=w495) -> (s? t:f=w493:dbl)
              n160 = Build Array(w449, w481, "堆芯反应性", w466, "堆芯反应性", w467, "堆芯反应性", w492, w491, nan ("元素")) -> (w520:dbl[])
              n161 = local write "输出电流 (A)"(w493) -> ()
              n162 = Build Array("VO 1", "VO 2", "VO 3", "VO 4") -> (w476:u16[])
              n163 = for {
                tunnel: w455 -> [w544]
                tunnel: [w545] -> w463 mode=indexing
                tunnel: "电压输出选择" -> [w546]
                tunnel: w476 -> [w542] mode=indexing
                n164 = Index Array(array=w544, index=w542) -> (element=w543:dbl)
                n165 = case shown="True" w546 {
                  tunnel: w543 -> [w549 w561]
                  tunnel: [w548 w560] -> w545
                  tunnel: w542 -> [w547 w559]
                  frame False {
                    n166 = case shown="Default" w547 {
                      tunnel: w549 -> [w551 w552 w554 w556 w558]
                      tunnel: [w550 w552 w553 w555 w557] -> w548
                      frame 5 {
                        # "硼浓度"
                        n167 = expression code="x*4/2000+1"(w551) -> (w550:dbl)
                      }
                      frame Default {
                      }
                      frame 7 {
                        # "源量程脉冲"
                        n168 = expression code="log(x)*4/7+1"(w554) -> (w553:dbl)
                      }
                      frame 6 {
                        # "中间量程电流"
                        n169 = expression code="(log(x)+11)/2+1"(w556) -> (w555:dbl)
                      }
                      frame 0..4 {
                        # "棒位"
                        n170 = expression code="x*4/225+1"(w558) -> (w557:dbl)
                      }
                    }
                  }
                  frame True {
                    n171 = case shown="0" w559 {
                      tunnel: w561 -> [w563 w565 w566 w568 w570 w572]
                      tunnel: [w562 w564 w566 w567 w569 w571] -> w560
                      frame 3 {
                        # "温度"
                        n172 = expression code="(x-275)*10/60"(w563) -> (w562:dbl)
                      }
                      frame 4 {
                        # "硼浓度"
                        n173 = expression code="x*10/2000"(w565) -> (w564:dbl)
                      }
                      frame Default {
                      }
                      frame 0 {
                        # "源量程脉冲"
                        n174 = expression code="log(x)*10/7"(w568) -> (w567:dbl)
                      }
                      frame 1 {
                        # "中间量程电流"
                        n175 = expression code="(log(x)+11)/0.8"(w570) -> (w569:dbl)
                      }
                      frame 2 {
                        # "棒位"
                        n176 = expression code="10*x/225"(w572) -> (w571:dbl)
                      }
                    }
                  }
                }
              }
              "输出电压" <- w463
              n177 = Array To Spreadsheet String(array=w520, 3:"%g" ("format string")) -> (spreadsheet string=w519:string)  [unwired: 1 in]
              n178 = Unbundle By Name(w475) -> ("status"=w474:bool)
              n179 = Not(x=w474) -> (.not. x?=w473:bool)
              n180 = And(x=w472, y=w473) -> (x .and. y?=w456:bool)
              n181 = local write "TCP服务器开关"(w456) -> ()
              n182 = Write to Text File(file (use dialog)=w524, text=w519, error in=w523) -> (refnum out=w522:refnum<file>, error out=w521:errorcluster)  [unwired: 1 in, 1 out]
              n183 = local read "退出"() -> (w459:bool)
            }
            n184 = Not Equal?(x=w59, y=w57) -> (x != y?=w78:bool)
            n185 = Not Equal?(x=w56, y=w57) -> (x != y?=w58:bool)
            n186 = Not Equal?(x=w55, y=w81) -> (x != y?=w82:bool)
            n187 = Not Equal?(x=w53, y=w81) -> (x != y?=w54:bool)
            n188 = case shown="True" w78 {
              tunnel: w59 -> [_ w330]
              frame False {
                n189 = property on="电流输出选择" class="Ring (strict)"("DisabledEnum"=T1."Disabled and Grayed Out" ("禁用")) -> ()  [unwired: 2 in, 2 out]
              }
              frame True {
                w322 = T7 {"Auto Range?"=TRUE, "Man / Selected\nRange"=enum."2nA"}  # Current Range In
                w329 = FALSE  # Check For SCPI Errors? (T)
                w326 = FALSE ("Read Back Set Values? (T)")
                n190 = call "Initialize.vi"("VISA resource name"=w330, "Error Queue Option"=enum16{"Clear Error Queue", "Error Query"}."Clear Error Queue", "Instrument Type"=KE622x_--_Instrument_Type."KE6220") -> ("VISA resource name out"=w320:refnum<visa-resource-name>, "error out"=w319:errorcluster)  [unwired: 11 in]
                n191 = property on="电流输出选择" class="Ring (strict)"("DisabledEnum"=T1."Enabled" ("禁用")) -> ()  [unwired: 2 in, 2 out]
                n192 = Boolean To (0,1)(Boolean=FALSE ("布尔")) -> (0, 1=w312:i16)
                n193 = call "KE622x -- Set Analog Filter State.vi"("Resource In"=w320, "Check For SCPI Errors? (T)"=w329, "Analog Filter State"=w312, "error in (no error)"=w319) -> ("Resource Out (dupl)"=w316:refnum<visa-resource-name>, "error out"=w317:errorcluster)  [unwired: 10 in]
                n194 = call "KE622x -- Set Current Range.vi"("Resource In"=w316, "Check For SCPI Errors? (T)"=w329, "Current Range In"=w322, "error in (no error)"=w317, "Read Back Set Values? (T)"=w326) -> ("Resource Out (dupl)"=w314:refnum<visa-resource-name>, "error out"=w313:errorcluster)  [unwired: 8 in, 1 out]
                n195 = call "KE622x -- Set Voltage Limit.vi"("Resource In"=w314, "Check For SCPI Errors? (T)"=w329, "Voltage Limit (V)"=T3 10.0, "error in (no error)"=w313) -> ("Resource Out (dupl)"=w328:refnum<visa-resource-name>, "error out"=w327:errorcluster)  [unwired: 10 in]
                n196 = while {
                  tunnel: w329 -> [w346]
                  tunnel: w328 -> [w345]
                  tunnel: w327 -> [w344]
                  tunnel: w326 -> [w343]
                  tunnel: [w342] -> w325
                  tunnel: [w341] -> w324
                  tunnel: [w336] -> w323
                  stop <- w333 stop-if-true
                  n197 = call "KE622x -- Set Current Level.vi"("Resource In"=w345, "Check For SCPI Errors? (T)"=w346, "Current Level (A) In"="输出电流 (A)", "error in (no error)"=w344, "Read Back Set Value? (T)"=w343) -> ("Resource Out (dupl)"=w340:refnum<visa-resource-name>, "error out"=w339:errorcluster)  [unwired: 8 in, 1 out]
                  n198 = Boolean To (0,1)(Boolean=TRUE ("布尔")) -> (0, 1=w338:i16)
                  n199 = case shown="0, Default" w338 {
                    selector: w338 -> [w350 _]
                    tunnel: w340 -> [w352 w358]
                    tunnel: w339 -> [w351 w357]
                    tunnel: [w349 w355] -> w336
                    tunnel: w346 -> [w347 w353]
                    tunnel: [w348 w354] -> w341
                    tunnel: [w347 w353] -> w342
                    frame 0, Default {
                      n200 = call "KE622x -- Set Output State.vi"("Resource In"=w352, "Check For SCPI Errors? (T)"=w347, "Output State"=w350, "error in (no error)"=w351) -> ("Resource Out (dupl)"=w348:refnum<visa-resource-name>, "error out"=w349:errorcluster)  [unwired: 10 in]
                    }
                    frame 1 {
                      n201 = call "KE622x -- Turn Output On And Check For Errors.vi"("Resource In"=w358, "Check For SCPI Errors? (T)"=w353, "Turn Off Output If Compliance?"=TRUE ("Turn Off Output\nIf Voltage Limit?"), "error in (no error)"=w357) -> ("Resource Out (dupl)"=w354:refnum<visa-resource-name>, "error out"=w355:errorcluster)  [unwired: 8 in, 2 out]
                    }
                  }
                  n202 = Unbundle By Name(w336) -> ("status"=w332:bool)
                  n203 = local read "停止"() -> (w334:bool)
                  n204 = Not(x=w332) -> (.not. x?=→"KE6220_1":bool)
                  n205 = Or(x=w334, y=w332) -> (x .or. y?=w333:bool)
                }
                n206 = call "Close.vi"("VISA resource name"=w324, "Query For SCPI Errors? (T)"=w325, "error in (no error)"=w323) -> ("error out"=w310:errorcluster)  [unwired: 12 in]
                n207 = call <vilib>:"Simple Error Handler.vi"("error in (no error)"=w310) -> ()  [unwired: 4 in, 5 out]
              }
            }
            n208 = case shown="True" w58 {
              tunnel: w56 -> [_ w128]
              frame False {
              }
              frame True {
                w120 = T7 {"Auto Range?"=TRUE, "Man / Selected\nRange"=enum."2nA"}  # Current Range In
                w127 = FALSE  # Check For SCPI Errors? (T)
                w124 = FALSE ("Read Back Set Values? (T)")
                n209 = call "Initialize.vi"("VISA resource name"=w128, "Error Queue Option"=enum16{"Clear Error Queue", "Error Query"}."Clear Error Queue", "Instrument Type"=KE622x_--_Instrument_Type."KE6220") -> ("VISA resource name out"=w118:refnum<visa-resource-name>, "error out"=w117:errorcluster)  [unwired: 11 in]
                n210 = Boolean To (0,1)(Boolean=FALSE ("布尔")) -> (0, 1=w110:i16)
                n211 = call "KE622x -- Set Analog Filter State.vi"("Resource In"=w118, "Check For SCPI Errors? (T)"=w127, "Analog Filter State"=w110, "error in (no error)"=w117) -> ("Resource Out (dupl)"=w114:refnum<visa-resource-name>, "error out"=w115:errorcluster)  [unwired: 10 in]
                n212 = call "KE622x -- Set Current Range.vi"("Resource In"=w114, "Check For SCPI Errors? (T)"=w127, "Current Range In"=w120, "error in (no error)"=w115, "Read Back Set Values? (T)"=w124) -> ("Resource Out (dupl)"=w112:refnum<visa-resource-name>, "error out"=w111:errorcluster)  [unwired: 8 in, 1 out]
                n213 = call "KE622x -- Set Voltage Limit.vi"("Resource In"=w112, "Check For SCPI Errors? (T)"=w127, "Voltage Limit (V)"=T3 10.0, "error in (no error)"=w111) -> ("Resource Out (dupl)"=w126:refnum<visa-resource-name>, "error out"=w125:errorcluster)  [unwired: 10 in]
                n214 = while {
                  tunnel: w127 -> [w144]
                  tunnel: w126 -> [w143]
                  tunnel: w125 -> [w142]
                  tunnel: w124 -> [w141]
                  tunnel: [w140] -> w123
                  tunnel: [w139] -> w122
                  tunnel: [w134] -> w121
                  stop <- w133 stop-if-true
                  n215 = local read "输出电流 (A)"() -> (w129:dbl)
                  n216 = call "KE622x -- Set Current Level.vi"("Resource In"=w143, "Check For SCPI Errors? (T)"=w144, "Current Level (A) In"=w129, "error in (no error)"=w142, "Read Back Set Value? (T)"=w141) -> ("Resource Out (dupl)"=w138:refnum<visa-resource-name>, "error out"=w137:errorcluster)  [unwired: 8 in, 1 out]
                  n217 = Boolean To (0,1)(Boolean=TRUE ("布尔")) -> (0, 1=w136:i16)
                  n218 = case shown="0, Default" w136 {
                    selector: w136 -> [w148 _]
                    tunnel: w138 -> [w150 w156]
                    tunnel: w137 -> [w149 w155]
                    tunnel: [w147 w153] -> w134
                    tunnel: w144 -> [w145 w151]
                    tunnel: [w146 w152] -> w139
                    tunnel: [w145 w151] -> w140
                    frame 0, Default {
                      n219 = call "KE622x -- Set Output State.vi"("Resource In"=w150, "Check For SCPI Errors? (T)"=w145, "Output State"=w148, "error in (no error)"=w149) -> ("Resource Out (dupl)"=w146:refnum<visa-resource-name>, "error out"=w147:errorcluster)  [unwired: 10 in]
                    }
                    frame 1 {
                      n220 = call "KE622x -- Turn Output On And Check For Errors.vi"("Resource In"=w156, "Check For SCPI Errors? (T)"=w151, "Turn Off Output If Compliance?"=TRUE ("Turn Off Output\nIf Voltage Limit?"), "error in (no error)"=w155) -> ("Resource Out (dupl)"=w152:refnum<visa-resource-name>, "error out"=w153:errorcluster)  [unwired: 8 in, 2 out]
                    }
                  }
                  n221 = Unbundle By Name(w134) -> ("status"=w132:bool)
                  n222 = local read "停止"() -> (w131:bool)
                  n223 = Not(x=w132) -> (.not. x?=→"KE6220_2":bool)
                  n224 = Or(x=w131, y=w132) -> (x .or. y?=w133:bool)
                }
                n225 = call "Close.vi"("VISA resource name"=w122, "Query For SCPI Errors? (T)"=w123, "error in (no error)"=w121) -> ("error out"=w108:errorcluster)  [unwired: 12 in]
                n226 = call <vilib>:"Simple Error Handler.vi"("error in (no error)"=w108) -> ()  [unwired: 4 in, 5 out]
              }
            }
            n227 = case shown="True" w82 {
              tunnel: w83 -> [_ w160]
              tunnel: w62 -> [_ w159]
              tunnel: w55 -> [_ w158]
              frame False {
              }
              frame True {
                n228 = call-poly "VISA Configure Serial Port"("VISA resource name"=w158, "timeout (10sec)"=u32 1500, "Enable Termination\nChar (T)"=FALSE ("Termination(T)"), "baud rate (9600)"=w159) -> ("VISA resource name out"=w165:refnum<visa-resource-name>, "error out"=w164:errorcluster)  [unwired: 5 in, 5 out]
                n229 = while {
                  tunnel: w165 -> [w185]
                  tunnel: w164 -> [w184]
                  tunnel: [w179] -> w162
                  tunnel: [w174] -> w161
                  tunnel: w160 -> [w178]
                  stop <- w173 stop-if-true
                  n230 = property class="Instr"(reference=w185, error in=w184) -> (reference out=w182:refnum<visa-resource-name>, error out=w183:errorcluster, "Serial Settings:Number of Bytes at Serial Port"=w169:u32)
                  n231 = Greater Or Equal?(x=w169, y=u32 6) -> (x >= y?=w167:bool)
                  n232 = case shown="True" w167 {
                    tunnel: w183 -> [w187 w199]
                    tunnel: w182 -> [w188 w198]
                    tunnel: [w187 w197] -> w181
                    tunnel: [w188 w196] -> w180
                    tunnel: w178 -> [_ w194]
                    tunnel: w169 -> [_ w195]
                    tunnel: [-1 w190] -> w177
                    frame False {
                    }
                    frame True {
                      n233 = VISA Read(VISA resource name=w198, byte count=w195, error in (no error)=w199) -> (VISA resource name out=w196:refnum<visa-resource-name>, read buffer=w193:string, error out=w197:errorcluster)  [unwired: 1 out]
                      n234 = for {
                        tunnel: w194 -> [w203] mode=indexing
                        tunnel: w193 -> [w204]
                        tunnel: [w201] -> w191
                        tunnel: [w200] -> w192
                        i -> [w201]
                        stop <- w200 stop-if-true
                        n235 = Search/Split String(string=w204, search string/char (-)=w203) -> (offset of match=w202:i32)  [unwired: 1 in, 2 out]
                        n236 = Greater Or Equal To 0?(x=w202) -> (x >= 0?=w200:bool)
                      }
                      n237 = Select(t=w191, s=w192, f=-1) -> (s? t:f=w190:i32)
                    }
                  }
                  n238 = local read "功率量程 (A)"() -> (w175:dbl)
                  n239 = case shown="0" w177 {
                    tunnel: [w206 w214 w216 w228] -> w174
                    tunnel: w180 -> [w205 w213 w219 w227]
                    tunnel: w181 -> [w206 w212 w217 w226]
                    tunnel: [w205 w211 w218 w229] -> w179
                    tunnel: w175 -> [_ w208 _ w225]
                    tunnel: "KEITHLEY INSTRUMENTS INC.,MODEL 6485,4084828,C01   Jun 23 2010 12:22:00//H\r" ("y") -> [_ _ w215 _]
                    frame -1, Default {
                    }
                    frame 0 {
                      n240 = To Single Precision Float(number=w208) -> (single precision float=w210:sgl)
                      n241 = call "Sti_Switch.vi"("Integer32"=0, "自定义浮点32"=w210) -> ("20B_StrOut"=w209:string)  [unwired: 9 in]
                      n242 = VISA Write(VISA resource name=w213, write buffer=w209, error in (no error)=w212) -> (VISA resource name out=w211:refnum<visa-resource-name>, error out=w214:errorcluster)  [unwired: 1 out]
                    }
                    frame 1 {
                      n243 = VISA Write(VISA resource name=w219, write buffer=w215, error in (no error)=w217) -> (VISA resource name out=w218:refnum<visa-resource-name>, error out=w216:errorcluster)  [unwired: 1 out]
                    }
                    frame 2 {
                      n244 = Number To Exponential String(number=w225, precision (6)=i16 6 ("精度(6)"), 3:i16 13 ("宽度(-)")) -> (E-format string=w222:string)  [unwired: 1 in]
                      n245 = Concatenate Strings(w222, "\r" ("字符串")) -> (w221:string)
                      n246 = VISA Write(VISA resource name=w227, write buffer=w221, error in (no error)=w226) -> (VISA resource name out=w229:refnum<visa-resource-name>, error out=w228:errorcluster)  [unwired: 1 out]
                    }
                  }
                  n247 = local read "停止"() -> (w172:bool)
                  n248 = Unbundle By Name(w174) -> ("status"=w171:bool)
                  n249 = Not(x=w171) -> (.not. x?=→"COM1":bool)
                  n250 = Or(x=w171, y=w172) -> (x .or. y?=w173:bool)
                }
                n251 = VISA Close(VISA resource name=w162, error in (no error)=w161) -> (error out=w163:errorcluster)
                n252 = call <vilib>:"Simple Error Handler.vi"("error in (no error)"=w163) -> ()  [unwired: 1 in, 8 out]
              }
            }
            n253 = case shown="True" w54 {
              tunnel: w83 -> [_ w232]
              tunnel: w53 -> [_ w231]
              tunnel: w62 -> [_ w230]
              frame False {
              }
              frame True {
                n254 = call-poly "VISA Configure Serial Port"("VISA resource name"=w231, "timeout (10sec)"=u32 1500, "Enable Termination\nChar (T)"=FALSE ("Termination(T)"), "baud rate (9600)"=w230) -> ("VISA resource name out"=w235:refnum<visa-resource-name>, "error out"=w236:errorcluster)  [unwired: 5 in, 5 out]
                n255 = while {
                  tunnel: w235 -> [w258]
                  tunnel: w236 -> [w257]
                  tunnel: [w252] -> w238
                  tunnel: [w247] -> w239
                  tunnel: w232 -> [w251]
                  stop <- w246 stop-if-true
                  n256 = property class="Instr"(reference=w258, error in=w257) -> (reference out=w255:refnum<visa-resource-name>, error out=w256:errorcluster, "Serial Settings:Number of Bytes at Serial Port"=w241:u32)
                  n257 = Greater Or Equal?(x=w241, y=u32 6) -> (x >= y?=w240:bool)
                  n258 = case shown="True" w240 {
                    tunnel: w256 -> [w260 w272]
                    tunnel: w255 -> [w261 w271]
                    tunnel: [w260 w270] -> w254
                    tunnel: [w261 w269] -> w253
                    tunnel: w251 -> [_ w267]
                    tunnel: w241 -> [_ w268]
                    tunnel: [-1 w263] -> w250
                    frame False {
                    }
                    frame True {
                      n259 = VISA Read(VISA resource name=w271, byte count=w268, error in (no error)=w272) -> (VISA resource name out=w269:refnum<visa-resource-name>, read buffer=w266:string, error out=w270:errorcluster)  [unwired: 1 out]
                      n260 = for {
                        tunnel: w267 -> [w276] mode=indexing
                        tunnel: w266 -> [w277]
                        tunnel: [w274] -> w264
                        tunnel: [w273] -> w265
                        i -> [w274]
                        stop <- w273 stop-if-true
                        n261 = Search/Split String(string=w277, search string/char (-)=w276) -> (offset of match=w275:i32)  [unwired: 1 in, 2 out]
                        n262 = Greater Or Equal To 0?(x=w275) -> (x >= 0?=w273:bool)
                      }
                      n263 = Select(t=w264, s=w265, f=-1) -> (s? t:f=w263:i32)
                    }
                  }
                  n264 = local read "中间量程 (A)"() -> (w248:dbl)
                  n265 = case shown="0" w250 {
                    tunnel: [w279 w287 w289 w301] -> w247
                    tunnel: w253 -> [w278 w286 w292 w300]
                    tunnel: w254 -> [w279 w285 w290 w299]
                    tunnel: [w278 w284 w291 w302] -> w252
                    tunnel: w248 -> [_ w281 _ w298]
                    tunnel: "KEITHLEY INSTRUMENTS INC.,MODEL 6485,4084828,C01   Jun 23 2010 12:22:00//H\r" ("y") -> [_ _ w288 _]
                    frame -1, Default {
                    }
                    frame 0 {
                      n266 = To Single Precision Float(number=w281) -> (single precision float=w283:sgl)
                      n267 = call "Sti_Switch.vi"("Integer32"=0, "自定义浮点32"=w283) -> ("20B_StrOut"=w282:string)  [unwired: 9 in]
                      n268 = VISA Write(VISA resource name=w286, write buffer=w282, error in (no error)=w285) -> (VISA resource name out=w284:refnum<visa-resource-name>, error out=w287:errorcluster)  [unwired: 1 out]
                    }
                    frame 1 {
                      n269 = VISA Write(VISA resource name=w292, write buffer=w288, error in (no error)=w290) -> (VISA resource name out=w291:refnum<visa-resource-name>, error out=w289:errorcluster)  [unwired: 1 out]
                    }
                    frame 2 {
                      n270 = Number To Exponential String(number=w298, precision (6)=i16 6 ("精度(6)"), 3:i16 13 ("宽度(-)")) -> (E-format string=w295:string)  [unwired: 1 in]
                      n271 = Concatenate Strings(w295, "\r" ("字符串")) -> (w294:string)
                      n272 = VISA Write(VISA resource name=w300, write buffer=w294, error in (no error)=w299) -> (VISA resource name out=w302:refnum<visa-resource-name>, error out=w301:errorcluster)  [unwired: 1 out]
                    }
                  }
                  n273 = local read "停止"() -> (w245:bool)
                  n274 = Unbundle By Name(w247) -> ("status"=w243:bool)
                  n275 = Not(x=w243) -> (.not. x?=→"COM2":bool)
                  n276 = Or(x=w243, y=w245) -> (x .or. y?=w246:bool)
                }
                n277 = VISA Close(VISA resource name=w238, error in (no error)=w239) -> (error out=w237:errorcluster)
                n278 = call <vilib>:"Simple Error Handler.vi"("error in (no error)"=w237) -> ()  [unwired: 1 in, 8 out]
              }
            }
            n279 = Close File(refnum=w38, error in=w37) -> ()  [unwired: 2 out]
            n280 = call-dynamic "Shutdown.vi"("error in"=w65, "Modbus slave in"=w64) -> ("error out"=w63:errorcluster)  [unwired: 9 in]
            n281 = call <vilib>:"Clear Errors.vi"("error in (no error)"=w63) -> ()  [unwired: 5 in, 2 out]
          }
          frame True {
            # "未开始时就关闭窗口，不执行任何代码，直接退出。"
          }
        }
      }
    }
  }
  n282 = call <vilib>:"Application Directory.vi"() -> ("Application Directory"=w15:path)
  n283 = Build Path(base path=w15, name or relative path="rodValue.txt") -> (appended path=w8:path)
  n284 = call-poly <vilib>:"Read Delimited Spreadsheet.vi"("file path (dialog if empty)"=w8) -> ("all rows"=w9:dbl[][])  [unwired: 9 in, 5 out]
  n285 = Delete From Array(array=w9, index (row)=0 ("索引 (行)")) -> (array with subset deleted=w1:dbl[][])  [unwired: 2 in, 1 out]
  n286 = call-poly <userlib>:"Reverse 2D Array__ogtk.vi"("Array"=w1) -> ("Reversed Array"=w2:dbl[][])  [unwired: 2 in]
  n287 = for {
    tunnel: w2 -> [w638] mode=indexing
    tunnel: [w636] -> w7 mode=indexing
    tunnel: [w632] -> w6 mode=indexing
    tunnel: [w631] -> w3 mode=indexing
    tunnel: [w630] -> w4 mode=indexing
    tunnel: [w628] -> w5 mode=indexing
    w629 = cluster{"x":dbl, "y":dbl} {"x"=0.0, "y"=0.0} ("输入簇")
    n288 = Index Array(array=w638) -> (element #1=w626:dbl, element #2=w637:dbl, element #3=w635:dbl, element #4=w634:dbl, element #5=w633:dbl, element #6=w627:dbl)  [unwired: 6 in]
    n289 = Bundle By Name(cluster=w629, "x"=w626, "y"=w637) -> (w636:cluster{"x":dbl, "y":dbl})
    n290 = Bundle By Name(cluster=w629, "x"=w626, "y"=w634) -> (w631:cluster{"x":dbl, "y":dbl})
    n291 = Bundle By Name(cluster=w629, "x"=w626, "y"=w635) -> (w632:cluster{"x":dbl, "y":dbl})
    n292 = Bundle By Name(cluster=w629, "x"=w626, "y"=w633) -> (w630:cluster{"x":dbl, "y":dbl})
    n293 = Bundle By Name(cluster=w629, "x"=w626, "y"=w627) -> (w628:cluster{"x":dbl, "y":dbl})
  }
  n294 = call <vilib>:"General Polynomial Fit.vi"("Y"=w20, "polynomial order"=2, "X"=w19) -> ("Polynomial Coefficients"=w17:dbl[])  [unwired: 9 in, 3 out]
  n295 = while {
    stop <- w639 stop-if-true
    n296 = event shown="[0] \"开始降棒\": Value Change" {
      selector: _ -> [_ _]
      dyn-events: _ -> [_ _]
      timeout: _ -> [_ _]
      tunnel: [_ TRUE ("停止")] -> w639
      event "开始降棒": Value Change {
        n297 = event-data() -> ("NewVal"=w640:bool)  [unwired: 1 in]
        n298 = case shown="True" w640 {
          frame False {
          }
          frame True {
            n299 = while {
              stop <- w641 stop-if-true
              n300 = Divide(x="棒速(step/min)", y=60000.0) -> (x/y=w648:dbl)
              n301 = Multiply(x="细分时间 (ms)", y=w648) -> (x*y=w647:dbl)
              n302 = Wait (ms)(milliseconds to wait="细分时间 (ms)") -> ()  [unwired: 1 out]
              n303 = case shown="0, Default" "降棒选择" {
                tunnel: w647 -> [w657 w661 w667 w673 w679]
                tunnel: [w654 w660 w666 w672 w678] -> w644
                frame 0, Default {
                  w655 = 0.0 ("y")
                  n304 = local read "D棒组"() -> (w658:dbl)
                  n305 = Subtract(x=w658, y=w657) -> (x-y=w656:dbl)
                  n306 = Greater?(x=w658, y=w655) -> (0:w654:bool)
                  n307 = Select(t=w656, s=w654, f=w655) -> (s? t:f=w653:dbl)
                  n308 = property on="D棒组" class="Slide (strict)"("Val(Sgnl)"=w653) -> ()  [unwired: 2 in, 2 out]
                }
                frame 1 {
                  w663 = 0.0 ("y")
                  n309 = local read "C棒组"() -> (w662:dbl)
                  n310 = Subtract(x=w662, y=w661) -> (x-y=w664:dbl)
                  n311 = Greater?(x=w662, y=w663) -> (0:w660:bool)
                  n312 = Select(t=w664, s=w660, f=w663) -> (s? t:f=w659:dbl)
                  n313 = property on="C棒组" class="Slide (strict)"("Val(Sgnl)"=w659) -> ()  [unwired: 2 in, 2 out]
                }
                frame 2 {
                  w669 = 0.0 ("y")
                  n314 = local read "B棒组"() -> (w668:dbl)
                  n315 = Subtract(x=w668, y=w667) -> (x-y=w670:dbl)
                  n316 = Greater?(x=w668, y=w669) -> (0:w666:bool)
                  n317 = Select(t=w670, s=w666, f=w669) -> (s? t:f=w665:dbl)
                  n318 = property on="B棒组" class="Slide (strict)"("Val(Sgnl)"=w665) -> ()  [unwired: 2 in, 2 out]
                }
                frame 3 {
                  w675 = 0.0 ("y")
                  n319 = local read "A棒组"() -> (w674:dbl)
                  n320 = Subtract(x=w674, y=w673) -> (x-y=w676:dbl)
                  n321 = Greater?(x=w674, y=w675) -> (0:w672:bool)
                  n322 = Select(t=w676, s=w672, f=w675) -> (s? t:f=w671:dbl)
                  n323 = property on="A棒组" class="Slide (strict)"("Val(Sgnl)"=w671) -> ()  [unwired: 2 in, 2 out]
                }
                frame 4 {
                  w682 = 0.0 ("y")
                  n324 = local read "S棒组"() -> (w680:dbl)
                  n325 = Subtract(x=w680, y=w679) -> (x-y=w681:dbl)
                  n326 = Greater?(x=w680, y=w682) -> (0:w678:bool)
                  n327 = Select(t=w681, s=w678, f=w682) -> (s? t:f=w677:dbl)
                  n328 = property on="S棒组" class="Slide (strict)"("Val(Sgnl)"=w677) -> ()  [unwired: 2 in, 2 out]
                }
              }
              n329 = local read "退出"() -> (w643:bool)
              n330 = Not(x="开始降棒") -> (.not. x?=w642:bool)
              n331 = case shown="False" w644 {
                frame False {
                  n332 = local write "开始降棒"(FALSE ("开始降棒")) -> ()
                }
                frame True {
                }
              }
              n333 = Or(x=w642, y=w643) -> (x .or. y?=w641:bool)
            }
          }
        }
      }
      event "退出": Value Change {
        n334 = event-data() -> ()  [unwired: 1 in, 6 out]
      }
    }
  }
  n335 = while {
    tunnel: w7 -> [w690]
    tunnel: w6 -> [w689]
    tunnel: w3 -> [w688]
    tunnel: w4 -> [w687]
    tunnel: w5 -> [w686]
    tunnel: w17 -> [w685]
    stop <- w684 stop-if-true
    n336 = event shown="[0] \"D棒组\", \"C棒组\", \"B棒组\", \"A棒组\", \"S棒组\", \"硼浓度 (ppm)\", \"堆芯后备反应性 (pcm)\": Value Change" {
      selector: _ -> [_ _ _ _ _ _ _]
      dyn-events: _ -> [_ _ _ _ _ _ _]
      timeout: _ -> [_ _ _ _ _ _ _]
      tunnel: w690 -> [w721 _ _ _ _ _ _]
      tunnel: w689 -> [w720 _ _ _ _ _ _]
      tunnel: w688 -> [w719 _ _ _ _ _ _]
      tunnel: w687 -> [w718 _ _ _ _ _ _]
      tunnel: w686 -> [w713 _ _ _ _ _ _]
      tunnel: w685 -> [w711 _ _ _ _ _ _]
      tunnel: [_ _ _ _ _ "退出" _] -> w684
      event "D棒组", "C棒组", "B棒组", "A棒组", "S棒组", "硼浓度 (ppm)", "堆芯后备反应性 (pcm)": Value Change {
        w712 = 1.0 ("x")
        # "插值X顺序必须为升序"
        n337 = event-data() -> ()  [unwired: 1 in, 6 out]
        n338 = call-poly <vilib>:"Polynomial Evaluation.vi"("P(x)"=w711, "a"="硼浓度 (ppm)") -> ("P(a)"=w710:dbl)  [unwired: 1 out]
        n339 = Interpolate 1D Array(1:"D棒组", 2:w721) -> (0:w706:dbl)
        "D棒价值" <- w706
        n340 = Interpolate 1D Array(1:"C棒组", 2:w720) -> (0:w705:dbl)
        "C棒价值" <- w705
        n341 = Interpolate 1D Array(1:"B棒组", 2:w719) -> (0:w704:dbl)
        "B棒价值" <- w704
        n342 = Interpolate 1D Array ("一维数组插值")(1:"S棒组", 2:w713) -> (0:w702:dbl)
        "S棒价值" <- w702
        n343 = Interpolate 1D Array(1:"A棒组", 2:w718) -> (0:w703:dbl)
        "A棒价值" <- w703
        n344 = Multiply(x=w710, y="硼浓度 (ppm)") -> (x*y=w691:dbl)
        "硼总价值 (pcm)" <- w691
        n345 = Build Array("硼浓度 (ppm)", "D棒组", "C棒组", "B棒组", "A棒组", "S棒组") -> (→"棒位与硼浓度":dbl[])
        n346 = Build Array(w706, w705, w704, w703, w702) -> (w717:dbl[])
        n347 = Add Array Elements(numeric array=w717) -> (sum=w692:dbl)
        "棒总价值 (pcm)" <- w692
        n348 = Add(x=w691, y=w692) -> (x+y=w707:dbl)
        n349 = Add(x=w707, y="堆芯后备反应性 (pcm)") -> (x+y=w694:dbl)
        "堆芯反应性(硼+棒) (pcm)" <- w694
        n350 = Multiply(x=1e-05, y=w694) -> (x*y=w715:dbl)
        n351 = Subtract(x=w712, y=w715) -> (x-y=w714:dbl)
        n352 = Divide(x=w712, y=w714) -> (x/y=→"keff":dbl)
        n353 = case shown="True" "反应性控制方式" {
          tunnel: w694 -> [_ w722]
          frame False {
          }
          frame True {
            n354 = local write "堆芯反应性"(w722) -> ()
          }
        }
        "硼浓度 indicator" <- "硼浓度 (ppm)"
      }
      event "归零": Value Change {
        n355 = event-data() -> ()  [unwired: 1 in, 6 out]
        n356 = disable-structure shown="Disabled" {
          frame Disabled {
            w728 = 0.0 ("堆芯反应性 (pcm)")
            n357 = local write "堆芯反应性(硼+棒) (pcm)"(w728) -> ()
            n358 = local write "堆芯反应性"(w728) -> ()
          }
          frame Enabled {
          }
        }
        n359 = local read "硼总价值 (pcm)"() -> (w725:dbl)
        n360 = local read "棒总价值 (pcm)"() -> (w724:dbl)
        n361 = Add(x=w725, y=w724) -> (x+y=w726:dbl)
        n362 = Subtract(x=0.0, y=w726) -> (x-y=w727:dbl)
        n363 = property on="堆芯后备反应性 (pcm)" class="DigNum (strict)"("Val(Sgnl)"=w727) -> ()  [unwired: 2 in, 2 out]
      }
      event "反应性控制方式": Value Change {
        n364 = event-data() -> ("NewVal"=w729:bool)  [unwired: 1 in, 5 out]
        n365 = case shown="True" w729 {
          frame False {
            n366 = property on="堆芯反应性" class="DigNum (strict)"("DisabledEnum"=T1."Enabled" ("Disabled")) -> ()  [unwired: 2 in, 2 out]
          }
          frame True {
            n367 = local read "堆芯反应性(硼+棒) (pcm)"() -> (w732:dbl)
            n368 = local write "堆芯反应性"(w732) -> ()
            n369 = property on="堆芯反应性" class="DigNum (strict)"("DisabledEnum"=T1."Disabled" ("Disabled")) -> ()  [unwired: 2 in, 2 out]
          }
        }
      }
      event "物理参数设置": Value Change {
        n370 = event-data() -> ()  [unwired: 1 in, 6 out]
        n371 = call "PhysicsDialog.vi"() -> ()  [unwired: 1 in]
      }
      event "电信号输出设置": Value Change {
        n372 = event-data() -> ()  [unwired: 1 in, 6 out]
        n373 = call "analogSettings.vi"() -> ()  [unwired: 12 in]
      }
      event "退出": Value Change {
        n374 = event-data() -> ()  [unwired: 1 in, 6 out]
        n375 = local write "停止"(TRUE ("停止")) -> ()
      }
      event Panel Close? {
        n376 = event-data() -> ()  [unwired: 1 in, 4 out]
        n377 = property on="退出" class="Bool (strict)"("Val(Sgnl)"=TRUE ("Value (Signaling)")) -> ()  [unwired: 2 in, 2 out]
        n378 = event-data("Discard?"=TRUE) -> ()  [unwired: 1 in, 1 out]
      }
    }
  }
